vi "push test data(com).vi"(8 "error in":errorcluster, 9 "rewrite/concatenate":bool=TRUE, 10 "array in":u8[][](array[numeric]) format="%x", 11 "VISA resource name in":refnum<visa-resource-name>) -> (0 "error out":errorcluster, 1 "return count":u32, 2 "transmitted array":u8[](array[numeric]), 3 "VISA resource name out":refnum<visa-resource-name>)   [LabVIEW 2017]
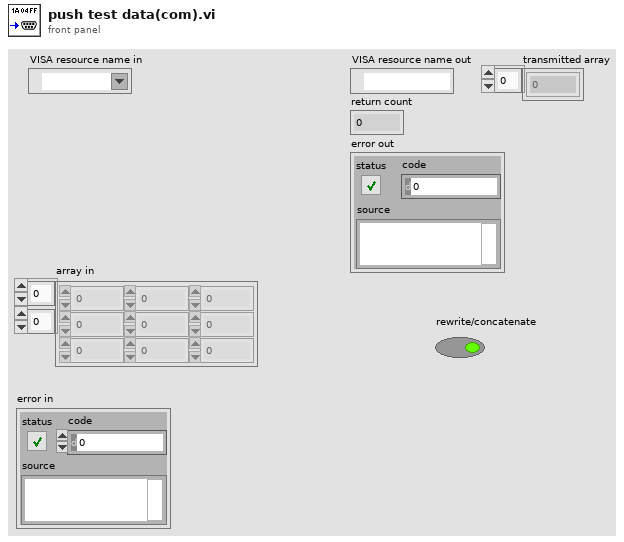
[diagram p1: front panel]
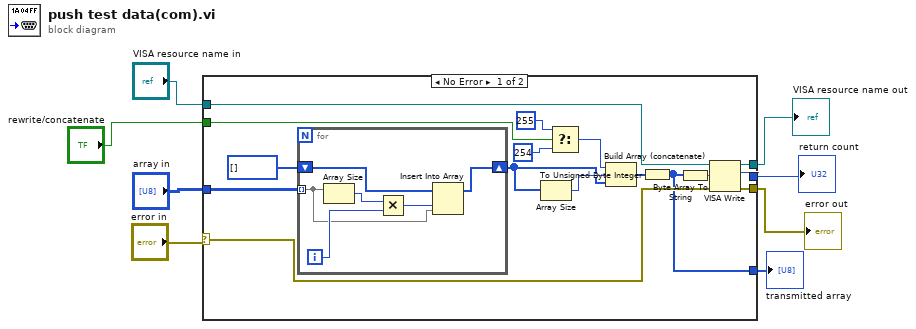
[diagram p0: block diagram]
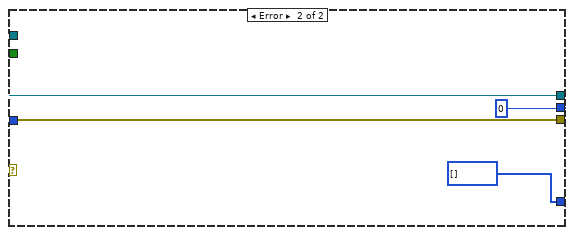
[diagram p2: hidden frame]
diagram:
  n1 = case shown="No Error" "error in" {
    selector: "error in" -> [w14 w34]
    tunnel: "array in" -> [w24 _]
    tunnel: "rewrite/concatenate" -> [w22 _]
    tunnel: "VISA resource name in" -> [w13 w33]
    tunnel: [w12 w33] -> w4
    tunnel: [w11 w34] -> w2
    tunnel: [w10 u32 0 ("return count")] -> w3
    tunnel: [w9 u8[] []] -> w1
    frame No Error {
      n2 = for {
        tunnel: w24 -> [w27] mode=indexing
        shift-right: [w25] -> w17
        shift-left: i32[] [] -> [w26]
        i -> [w30]
        n3 = Array Size(array=w27) -> (size(s)=w29:i32)
        n4 = Multiply(x=w29, y=w30) -> (x*y=w28:i32)
        n5 = Insert Into Array(array=w26, index=w28, new element=w27) -> (w25:i32[])
      }
      n6 = Array Size(array=w17) -> (size(s)=w18:i32)
      n7 = Select(t=u8 255, s=w22, f=u8 254) -> (s? t:f=w19:u8)
      n8 = Build Array (concatenate)(w19, w18, w17) -> (w16:i32[])
      n9 = To Unsigned Byte Integer(number=w16) -> (unsigned 8bit integer=w9:u8[])
      n10 = Byte Array To String(unsigned byte array=w9) -> (string=w15:string)
      n11 = VISA Write(VISA resource name=w13, write buffer=w15, error in (no error)=w14) -> (VISA resource name out=w12:refnum<visa-resource-name>, return count=w10:u32, error out=w11:errorcluster)
    }
    frame Error {
    }
  }
  "VISA resource name out" <- w4
  "return count" <- w3
  "error out" <- w2
  "transmitted array" <- w1
